vi "EncodeData.vi"(8 "error in (no error)":errorcluster, 9 "Secret":string, 10 "Data to Encode":variant, 11 "CryptoType":refnum<class "Crypto.AES.lvclass">) -> (0 "error out":errorcluster, 2 "Encoded Data":string)   [LabVIEW 2016, in "Crypto.AES.lvclass"]
uses:
  Crypto.AES.lvclass
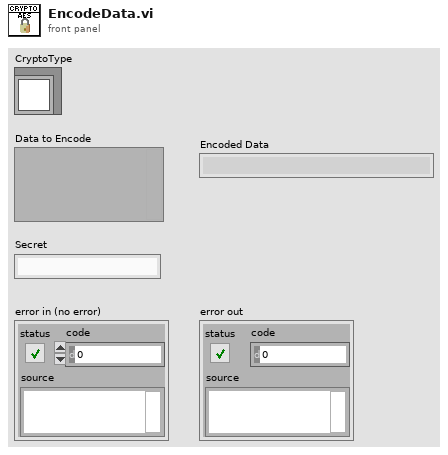
[diagram p1: front panel]
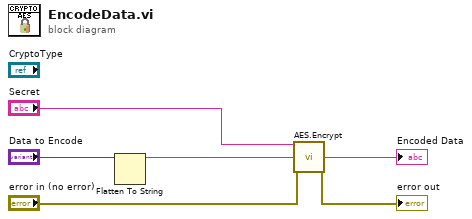
[diagram p0: block diagram]
diagram:
  n1 = Flatten To String(anything="Data to Encode") -> (data string=w1:string)  [unwired: 3 in, 2 out]
  n2 = call <vilib>:"AES.Encrypt.vi"("Password"="Secret", "PlainText"=w1, "error in"="error in (no error)") -> ("CypheredText"=→"Encoded Data":string, "error out"=→"error out":errorcluster)  [unwired: 11 in]
